vi "deactivateHWUserLED.vi"(8 "error in (no error)":errorcluster, 11 "Model in":refnum<class "Model.lvclass">) -> (0 "error out":errorcluster, 3 "Model out":refnum<class "Model.lvclass">)   [LabVIEW 2012, in "Model.lvclass"]
doc: "Turns off the hardware user LED."
uses:
  Model.lvclass
  Model.lvclass/Model.ctl
  Target/Target/Target.lvclass
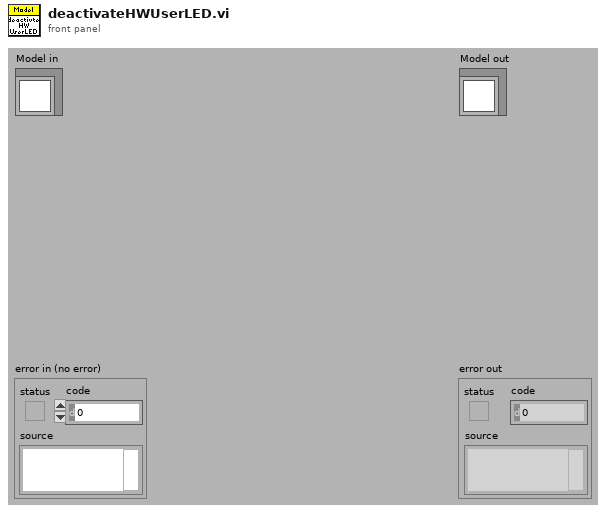
[diagram p1: front panel]
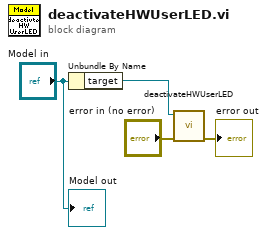
[diagram p0: block diagram]
diagram:
  n1 = Unbundle By Name("Model in") -> ("target"=w4:refnum<class "Target.lvclass">)
  n2 = call-dynamic "deactivateHWUserLED.vi"("error in (no error)"="error in (no error)", "Target in"=w4) -> ("error out"=→"error out":errorcluster)  [unwired: 8 in, 1 out]
  "Model out" <- "Model in"
